vi "Day7.vi"(11 "Input":string="190: 10 19\n3267: 81 40 27\n83: 17 5\n156: 15 6\n7290: 6 8 6 15\n161011: 16 10 13\n192: 17 8 14\n21037: 9 7 18 13\n292: 11 6 16 20") -> (3 "Result":i64)   [LabVIEW 2024]
uses:
  <vilib>/Utility/error.llb/Trim Whitespace One-Sided.vi
panel:
  out "Answers":i64[](array[numeric])
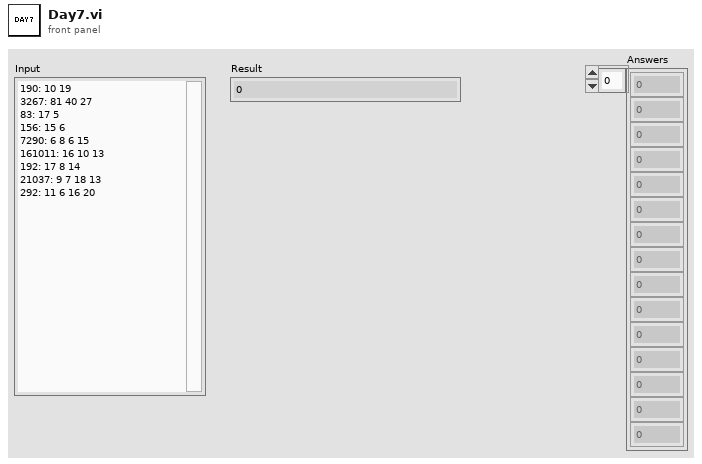
[diagram p1: front panel]
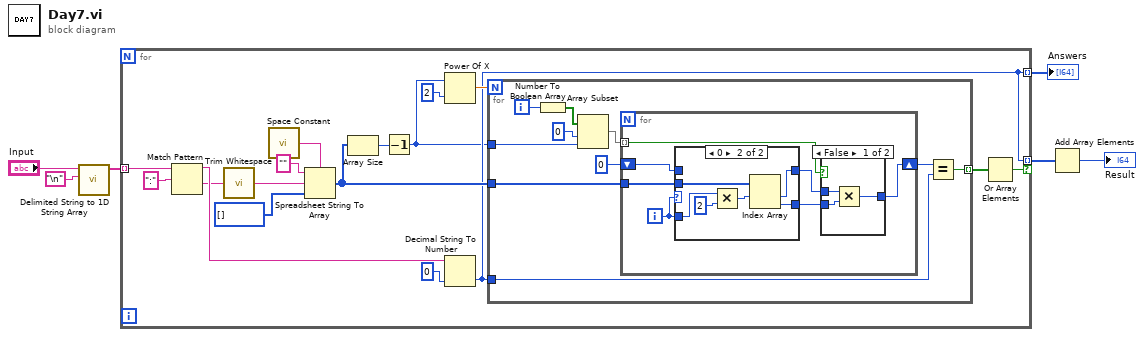
[diagram p0: block diagram]
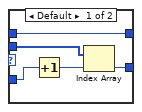
[diagram p2: hidden frame]
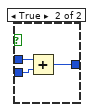
[diagram p3: hidden frame]
diagram:
  n1 = call <vilib>:"Delimited String to 1D String Array.vi"("delimiter"="\n", "delimited string"="Input") -> ("string array"=w4:string[])  [unwired: 9 in]
  n2 = for {
    tunnel: w4 -> [w23] mode=indexing
    tunnel: [w10] -> w3 mode=indexing
    tunnel: [w10] -> w2 mode=indexing if=w8
    n3 = Match Pattern(string=w23, regular expression=":") -> (before substring=w21:string, after substring=w20:string)  [unwired: 1 in, 2 out]
    n4 = call <vilib>:"Trim Whitespace.vi"("string"=w20) -> ("trimmed string"=w19:string)  [unwired: 1 in]
    n5 = call <vilib>:"Space Constant.vi"() -> ("String"=w17:string)
    n6 = Spreadsheet String To Array(delimiter (Tab)=w17, format string="", spreadsheet string=w19, array type (2D Dbl)=i64[] []) -> (array=w13:i64[])
    n7 = Array Size(array=w13) -> (size(s)=w14:i32)
    n8 = Decrement(x=w14) -> (x-1=w7:i32)
    n9 = Power Of X(1:2 ("y"), 2:w7) -> (0:w12:dbl)
    n10 = Decimal String To Number(string=w21, default (0L)=i64 0 ("default (0 I32)")) -> (number=w10:i64)  [unwired: 1 in, 1 out]
    n11 = for {
      N: w12 -> [_]
      tunnel: w13 -> [w32]
      tunnel: w10 -> [w29]
      tunnel: [w28] -> w9 mode=indexing
      tunnel: w7 -> [w24]
      i -> [w33]
      n12 = Number To Boolean Array(number=w33) -> (Boolean array=w27:bool[])
      n13 = Array Subset(array=w27, index=0, length=w24) -> (w26:bool[])
      n14 = for {
        tunnel: w32 -> [w40]
        tunnel: w26 -> [w39] mode=indexing
        shift-right: [w36] -> w30
        shift-left: i64 0 -> [w35]
        i -> [w34]
        n15 = case shown="0" w34 {
          tunnel: w40 -> [w45 w51]
          tunnel: [w43 w50] -> w38
          tunnel: [w44 w49] -> w37
          tunnel: w35 -> [w43 _]
          tunnel: w34 -> [w42 w47]
          frame Default {
            n16 = Increment(x=w42) -> (x+1=w41:i32)
            n17 = Index Array(array=w45, index=w41) -> (element=w44:i64)
          }
          frame 0 {
            n18 = Multiply(x=w47, y=2) -> (x*y=w46:i32)
            n19 = Index Array(array=w51, index #1=w46) -> (element #1=w50:i64, element #2=w49:i64)  [unwired: 1 in]
          }
        }
        n20 = case shown="False" w39 {
          tunnel: w38 -> [w54 w56]
          tunnel: w37 -> [w53 w57]
          tunnel: [w52 w55] -> w36
          frame False {
            n21 = Multiply(x=w54, y=w53) -> (x*y=w52:i64)
          }
          frame True {
            n22 = Add(x=w56, y=w57) -> (x+y=w55:i64)
          }
        }
      }
      n23 = Equal?(x=w30, y=w29) -> (x = y?=w28:bool)
    }
    n24 = Or Array Elements(Boolean array=w9) -> (logical OR=w8:bool)
  }
  "Answers" <- w3
  n25 = Add Array Elements(numeric array=w2) -> (sum=→"Result":i64)
